vi "Write MCListbox Refnum.vi"(8 "error in (no error)":errorcluster, 10 "MCListbox Refnum":refnum<vi>, 11 "MCLB_Lib in":refnum<class "MCLB_Lib.lvclass">) -> (0 "error out":errorcluster, 3 "MCLB_Lib out":refnum<class "MCLB_Lib.lvclass">)   [LabVIEW 2020]
uses:
  MCLB_Lib.lvclass
  MCLB_Lib.lvclass/MCLB_Lib.ctl
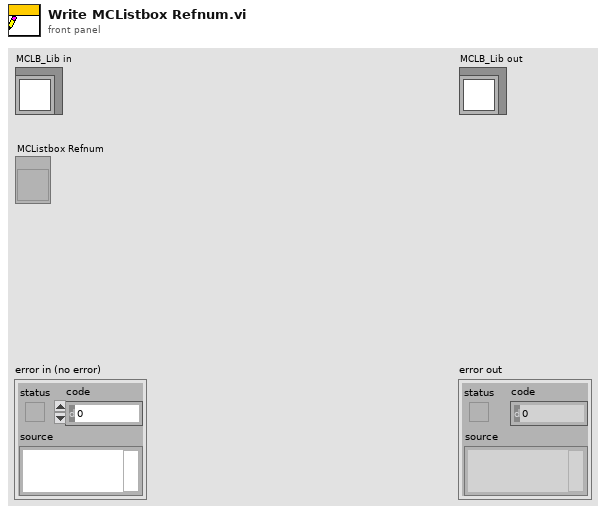
[diagram p1: front panel]
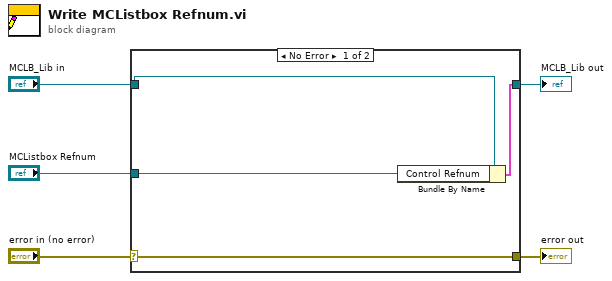
[diagram p0: block diagram]
diagram:
  n1 = case shown="No Error" "error in (no error)" {
    selector: "error in (no error)" -> [w9 w10]
    tunnel: [w9 w10] -> w4
    tunnel: [w7 w11] -> w2
    tunnel: "MCLB_Lib in" -> [w8 w11]
    tunnel: "MCListbox Refnum" -> [w6 _]
    frame No Error {
      n2 = Bundle By Name(cluster=w8, "Control Refnum"=w6) -> (w7:cluster{})
    }
    frame Error {
    }
  }
  "error out" <- w4
  "MCLB_Lib out" <- w2
